vi "load_image(SubVI).vi"(8 "error in (no error)":errorcluster, 11 "Image Path":path) -> (0 "error out":errorcluster, 3 "Image GRAY":T1)   [LabVIEW 2020]
doc: "Carica un'immagine dal percorso scelto. Restituisce un'immagine in formato RGB e un'immagine in bianco e nero tramite un cast."
uses:
  <vilib>/vision/Image Controls.llb/IMAQ Image.ctl
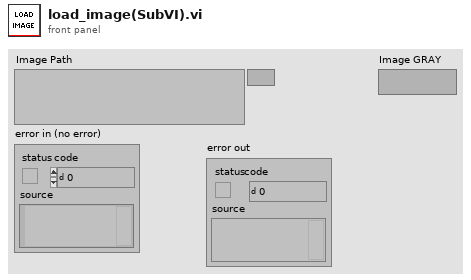
[diagram p1: front panel]
types:
  T1 = typedef "IMAQ Image.ctl" = refnum<image>
  T2 = typedef "Image Type" = u32
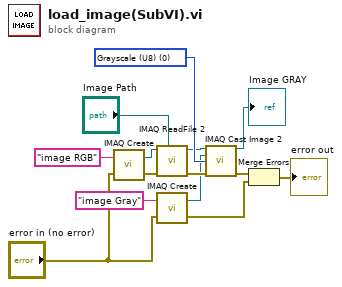
[diagram p0: block diagram]
diagram:
  w10 = T2 0 items=["Grayscale (U8)", "Grayscale (I16)", "Grayscale (SGL)", "Complex (CSG)", "RGB (U32)", "HSL (U32)", "RGB (U64)", "Grayscale (U16)"] ("Image Type")
  n1 = call "IMAQ Create"("Image Name"="image RGB", "error in (no error)"="error in (no error)") -> ("New Image"=w12:T1, "error out"=w13:errorcluster)  [unwired: 3 in]
  n2 = call "IMAQ ReadFile 2"("File Path"="Image Path", "error in (no error)"=w13, "Image"=w12) -> ("error out"=w9:errorcluster, "Image Out"=w1:T1)  [unwired: 4 in, 3 out]
  n3 = call "IMAQ Create"("Image Name"="image Gray", "error in (no error)"="error in (no error)") -> ("New Image"=w6:T1, "error out"=w4:errorcluster)  [unwired: 3 in]
  n4 = call "IMAQ Cast Image 2"("Image Src"=w1, "Image Dst"=w6, "Image Type"=w10, "error in (no error)"=w9) -> ("Image Dst Out"=→"Image GRAY":T1, "error out"=w3:errorcluster)  [unwired: 10 in]
  n5 = Merge Errors(w3, w4) -> (→"error out":errorcluster)
